vi "SaveDataFile.vi"(0 "Data Array":dbl[][](array[numeric]), 1 "Temperature":dbl, 2 "Run uninterrupted?":bool, 3 "Humidity":dbl, 7 "Sensor Index/\nSegment No.":u32, 11 "Error In":errorcluster, 12 "Array Titles":string, 13 "Strip Segment":string, 14 "Arrays format":string) -> (4 "Filename OUT":string, 6 "Pathname OUT":string, 10 "Path + Filename OUT":string, 15 "Error Out":errorcluster)   [LabVIEW 2013]
uses:
  globals/QC_RunInformation.vi
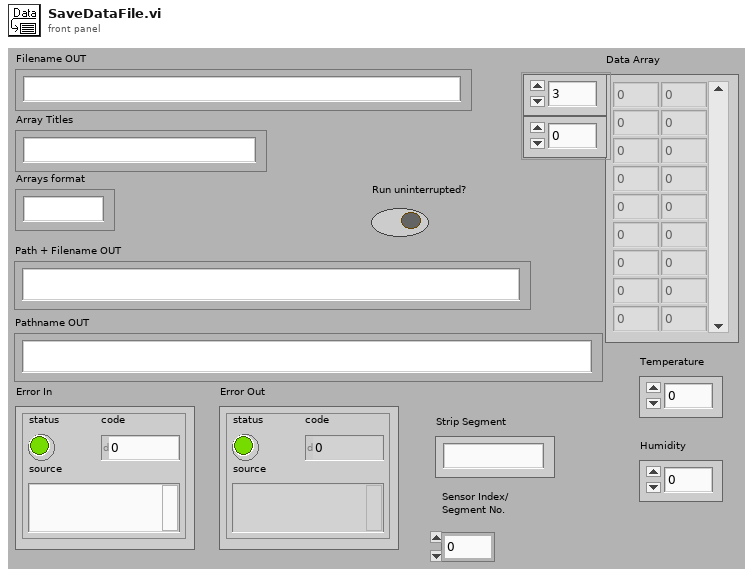
[diagram p1: front panel]
types:
  T1 = enum16{"open", "open or create", "create or replace", "create"}
  T2 = cluster{"Sensor Serial No.:":string, "Wafer:":string, "Batch:":string, "Manufacturer:":string, "Device Category:":string, "Database Serial No.:":string, "Date Initiated:":string, "Time Initiated:":string, "Test":string, "Probeplan used:":string, "End of Run comment:":string, "User:":string, "Vbias SMU":string, "LCR":string, "Test SMU":string, "Test DMM":string}
  T3 = cluster{"Institute":string, "Manufacturers":string[], "Devices":string[], "Serialnumbers Lookup DB":string, "Data directory":string, "Backup & screenshot directory":string, "List of known users":string[], "Measurement switch not used":bool, "Measurement Switch":string, "DUT Switch":string, "Rseries IV [MOhm]":string, "Rshunt IV [MOhm]":string, "Rseries CV [MOhm]":string, "DC blocking Cap [µF]":string, "Rseries LCR [MOhm]":string, "Rseries stability [MOhm]":string, "Rshunt stability [MOhm]":string, "Rseries striptest bias [MOhm]":string, "Rseries strip pinhole [MOhm]":string}
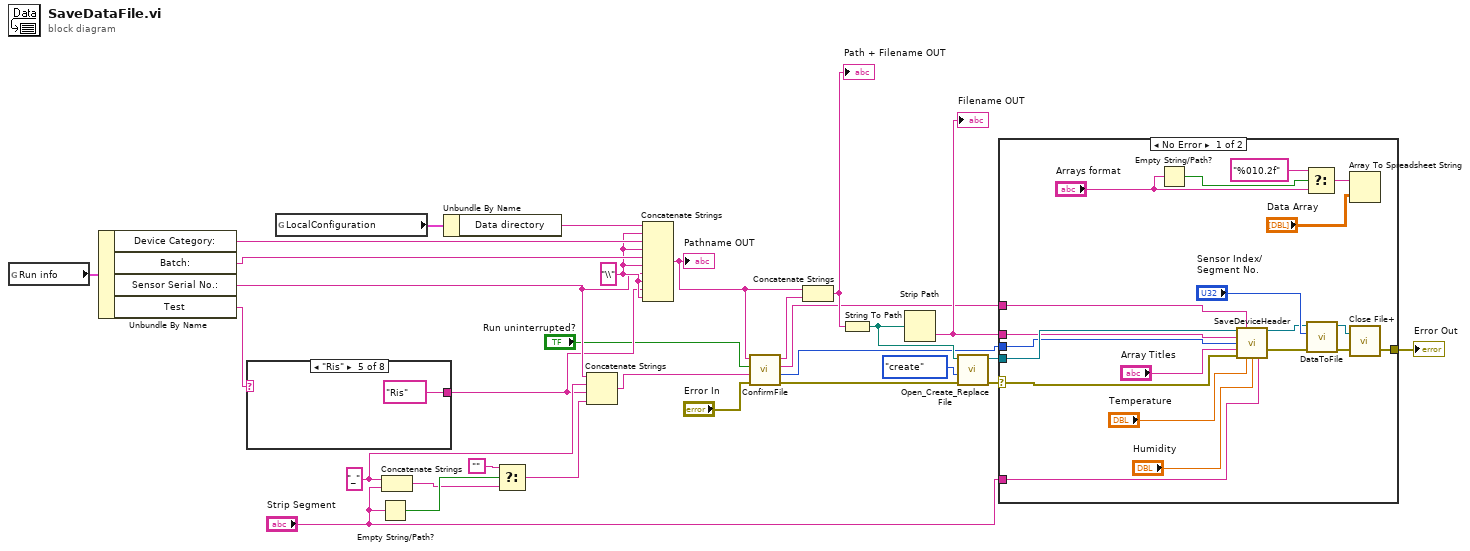
[diagram p0: block diagram]
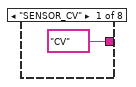
[diagram p2: hidden frame]
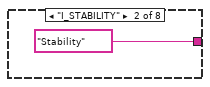
[diagram p3: hidden frame]
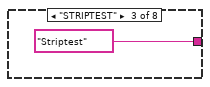
[diagram p4: hidden frame]
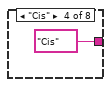
[diagram p5: hidden frame]
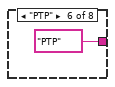
[diagram p6: hidden frame]
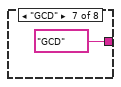
[diagram p7: hidden frame]
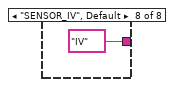
[diagram p8: hidden frame]
diagram:
  w10 = "_"
  w20 = "\\"
  n1 = global read "QC_RunInformation.vi" "Run info"() -> (w29:T2)
  n2 = Unbundle By Name(w29) -> ("Device Category:"=w27:string, "Batch:"=w26:string, "Sensor Serial No.:"=w7:string, "Test"=w4:string)
  n3 = case shown="\"Ris\"" w4 {
    tunnel: ["CV" ("Test") "Stability" ("Test") "Striptest" ("Test") "Cis" ("Test") "Ris" ("Test") "PTP" ("Test") "GCD" ("Test") "IV" ("Test")] -> w3
    frame "SENSOR_CV" {
    }
    frame "I_STABILITY" {
    }
    frame "STRIPTEST" {
    }
    frame "Cis" {
    }
    frame "Ris" {
    }
    frame "PTP" {
    }
    frame "GCD" {
    }
    frame "SENSOR_IV", Default {
    }
  }
  n4 = global read "QC_RunInformation.vi" "LocalConfiguration"() -> (w30:T3)
  n5 = Empty String/Path?(string/path="Strip Segment") -> (empty?=w12:bool)
  n6 = Concatenate Strings(w10, "Strip Segment") -> (w8:string)
  n7 = Unbundle By Name(w30) -> ("Data directory"=w28:string)
  n8 = Select(t="", s=w12, f=w8) -> (s? t:f=w9:string)
  n9 = Concatenate Strings(w7, w10, w3, w9) -> (w19:string)
  n10 = Concatenate Strings(w28, w20, w27, w20, w26, w20, w7, w20, w3, w20) -> (w15:string)
  "Pathname OUT" <- w15
  n11 = call "ConfirmFile.vi"("Error In"="Error In", "Filename IN"=w19, "Run uninterrupted?"="Run uninterrupted?", "Pathname IN"=w15) -> ("Error Out"=w16:errorcluster, "Run Number"=w6:i32, "comments OUT"=w1:string, "Filename:"=w14:string)
  n12 = Concatenate Strings(w15, w14) -> (w13:string)
  "Path + Filename OUT" <- w13
  n13 = String To Path(string=w13) -> (path=w22:path)
  n14 = Strip Path(path=w22) -> (name=w23:string)  [unwired: 1 out]
  "Filename OUT" <- w23
  n15 = call <vilib>:"Open_Create_Replace File.vi"("error in (no error)"=w16, "function (open:0)"=T1."create", "file path"=w22) -> ("error out"=w21:errorcluster, "refnum"=w24:refnum<file>)  [unwired: 5 in, 2 out]
  n16 = case shown="No Error" w21 {
    selector: w21 -> [w58 w59]
    tunnel: w24 -> [w52 _]
    tunnel: w23 -> [w51 _]
    tunnel: [w49 w59] -> w18
    tunnel: w6 -> [w46 _]
    tunnel: "Strip Segment" -> [w45 _]
    tunnel: w1 -> [w39 _]
    frame No Error {
      n17 = Empty String/Path?(string/path="Arrays format") -> (empty?=w55:bool)
      n18 = call "SaveDeviceHeader.vi"("File Refnum in"=w52, "Comments"=w39, "Filename"=w51, "Run Number"=w46, "Array Titles"="Array Titles", "error in (no error)"=w58, "Temperature"="Temperature", "Humidity"="Humidity", "Strip Segment"=w45) -> ("File Refnum out"=w43:refnum<file>, "error out"=w42:errorcluster)  [unwired: 4 in, 1 out]
      n19 = Select(t="%010.2f", s=w55, f="Arrays format") -> (s? t:f=w53:string)
      n20 = call "DataToFile.vi"("error in (no error)"=w42, "Sensor Index/\nSegment No."="Sensor Index/\nSegment No.", "File Refnum in"=w43) -> ("error out"=w41:errorcluster, "File Refnum out"=w40:refnum<file>)  [unwired: 7 in]
      n21 = Array To Spreadsheet String(array="Data Array", 3:w53) -> ()  [unwired: 1 in, 1 out]
      n22 = call <vilib>:"Close File+.vi"("error in (no error)"=w41, "refnum"=w40) -> ("error out"=w49:errorcluster)  [unwired: 3 in, 2 out]
    }
    frame Error {
    }
  }
  "Error Out" <- w18
